vi "Convert_UI_Laundry_ERD.vi"(0 "New Header?":bool, 2 "ERD Name":string[](array[string]), 5 "All_ERD_Data_Bundled_Brass In":T1, 7 "Array":T14[](array[typedef]) {"ERD Number" format="%.0x"}, 11 "Error In":errorcluster) -> (6 "All_ERD_Data_Bundled_Brass":T1, 15 "Error Out":errorcluster)   [LabVIEW 2021]
doc: "This VI parses the data from ERDs in correct format, units, etc. It handles all hex to dec conversions, hex to enum, and hex to boolean conversions.\n\nIf Raw Data from ERD is blank string, then it will output values from shift register."
uses:
  Common/LabVIEW GEA2 Toolkit/GEA3/type defs/ERD Read Data Out.ctl
  type defs/All_Bundled_Data.ctl
  type defs/Version.ctl
  type defs/ERD_Always_Show.ctl
  type defs/Brass Matrix.ctl
  type defs/CSV_File_String_Arrays.ctl
  type defs/Redundant.ctl
  type defs/Algorithms.ctl
  type defs/ATC_Data.ctl
  type defs/Fault Table Array.ctl
  type defs/Fault_Table_Info.ctl
  Dryer Tool (Commercial 2)/JL Dryer Tool Support/type defs/ERD_RJ45.ctl
  Dryer Tool (Commercial 2)/JL Dryer Tool Support/type defs/ERD_Commercial_Laundry.ctl
  type defs/BootloaderVersion.ctl
panel:
  out "ERD Number":u16 format="%x"
  # "Wet Load Size"
  # "Dry Load Size"
  # "OOB"
  # "Wet Load Size"
  # "Dry Load Size"
  # "OOB"
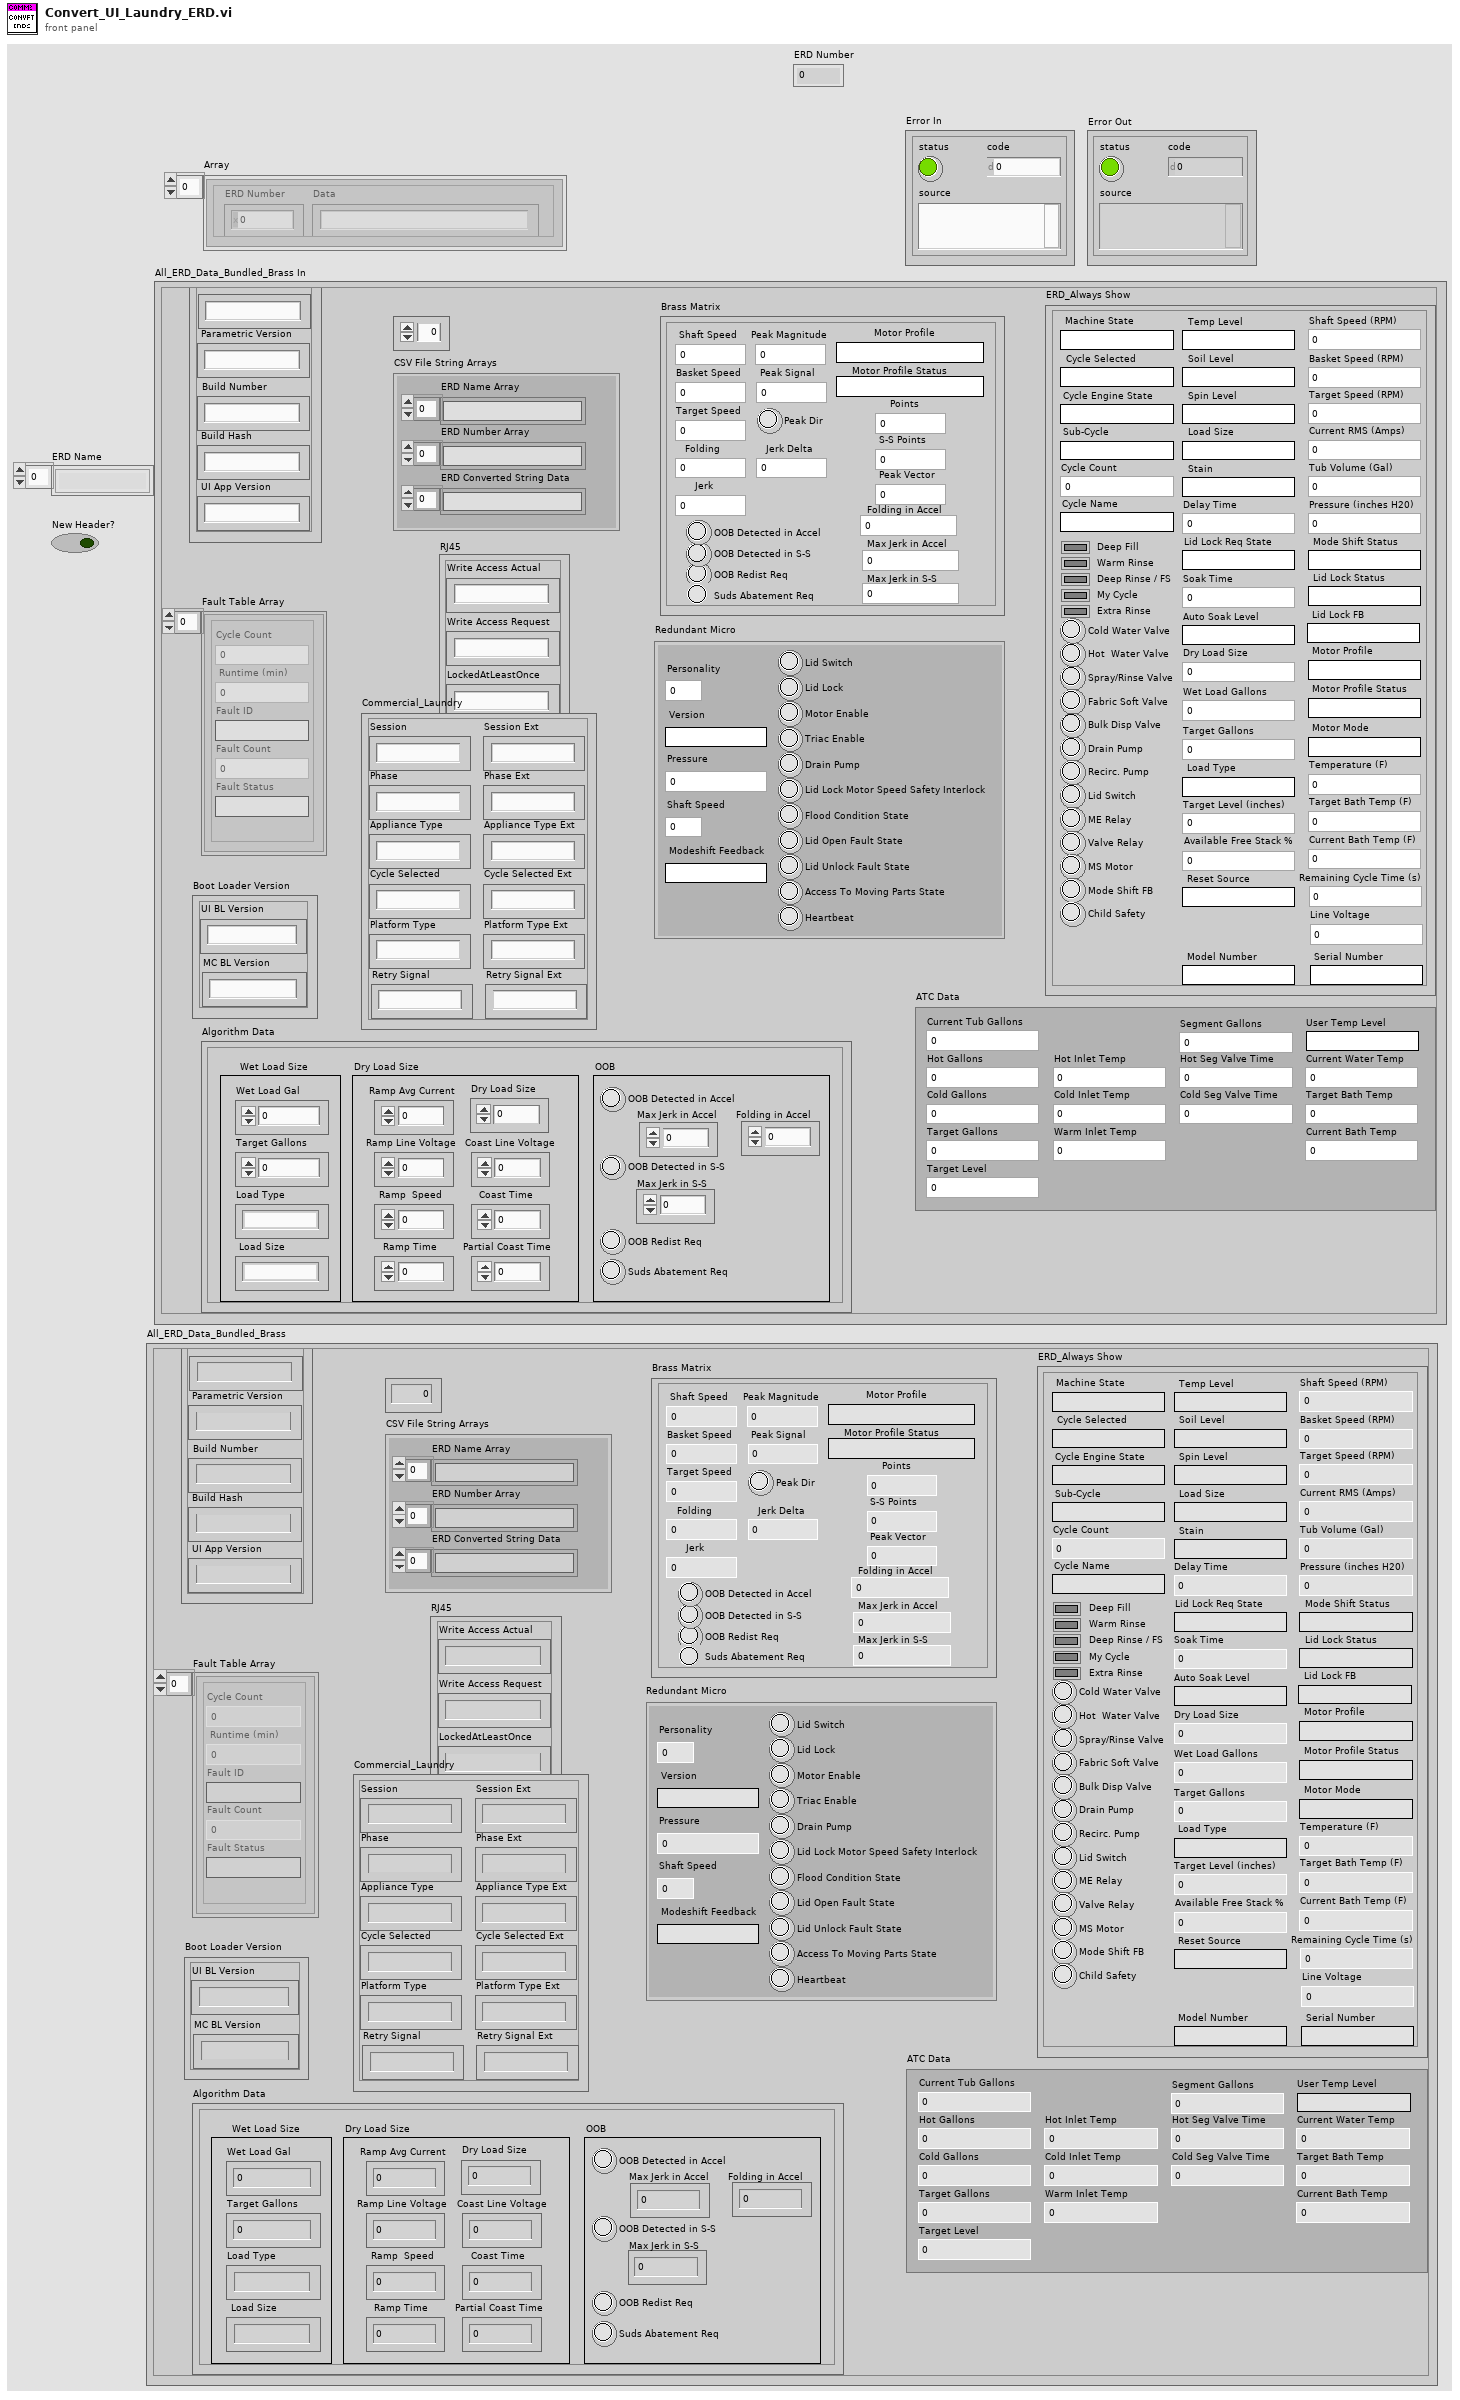
[diagram p1: front panel]
types:
  T1 = typedef "All_Bundled_Data.ctl" = cluster{"Software MC":T2, "ERD_Always Show":T3, "Personality Set":u8, "Brass Matrix":T4, "CSV File String Arrays":T5, "Redundant Micro":T6, "Algorithm Data":T7, "ATC Data":T8, "Fault Table Array ":T9, "RJ45":T11, "Commercial_Laundry":T12, "Boot Loader Version":T13}
  T2 = typedef "Version.ctl" = cluster{"Build Number":string, "Build Hash ":string, "Application Version":string, "Parametric Version":string, "UI App Version":string}
  T3 = typedef "ERD_Always_Show.ctl" = cluster{"Basket Speed (RPM)":u16, "Machine State":string, "Tub Volume (Gal)":dbl, "Pressure (inches H20)":dbl, "Lid Switch ":bool, "Current RMS (Amps)":dbl, "Cycle Selected":string, "Lid Lock Status":string, "Mode Shift Status":string, "Spray/Rinse Valve":bool, "Fabric Soft Valve":bool, "Drain Pump":bool, "Recirc. Pump":bool, "Cycle Engine State":string, "Hot  Water Valve":bool, "Cold Water Valve":bool, "Motor Profile":string, "Motor Profile Status":string, "Motor Mode":string, "ME Relay":bool, "Cycle Count":u32, "Deep Rinse / FS":bool, "My Cycle":bool, "Soil Level":string, "Spin Level":string, "Stain":string, "Temp Level":string, "Load Size":string, "Delay Time":u16, "Soak Time":u16, "Deep Fill":bool, "Warm Rinse":bool, "Auto Soak Level":string, "Extra Rinse":bool, "Wet Load Gallons":dbl, "Target Gallons":dbl, "Sub-Cycle":string, "Load Type":string, "Target Level (inches)":dbl, "Valve Relay":bool, "Dry Load Size":dbl, "Shaft Speed (RPM) ":u16, "MS Motor":bool, "Mode Shift FB":bool, "Target Bath Temp (F)":dbl, "Temperature (F)":dbl, "Current Bath Temp (F)":dbl, "Lid Lock FB":string, "Lid Lock Req State":string, "Remaining Cycle Time (s)":u32, "Available Free Stack %":u8, "Child Safety":bool, "Target Speed (RPM)":u16, "Reset Source":string, "Line Voltage":dbl, "Cycle Name":string, "Bulk Disp Valve":bool, "Model Number":string, "Serial Number":string}
  T4 = typedef "Brass Matrix.ctl" = cluster{"Shaft Speed":u16, "Folding":i32, "Jerk":i32, "Basket Speed":u16, "Target Speed":u16, "Peak Signal":u8, " Peak Magnitude":dbl, "Folding in Accel":i32, "Max Jerk in Accel":i32, "Max Jerk in S-S":i32, "Motor Profile Status":string, "Motor Profile":string, "OOB Redist Req":bool, "OOB Detected in S-S":bool, "OOB Detected in Accel":bool, "Suds Abatement Req ":bool, "Peak Dir":bool, "Peak Vector":dbl, "S-S Points":u8, "Points":u8, "Jerk Delta":i32}
  T5 = typedef "CSV_File_String_Arrays.ctl" = cluster{"ERD Number Array":string[], "ERD Name Array":string[], "ERD Converted String Data":string[]}
  T6 = typedef "Redundant.ctl" = cluster{"Version":string, "Personality":u8, "Pressure ":dbl, "Shaft Speed":u16, "Modeshift Feedback":string, "Lid Switch":bool, "Lid Lock":bool, "Triac Enable":bool, "Drain Pump":bool, "Lid Lock Motor Speed Safety Interlock":bool, "Flood Condition State":bool, "Lid Open Fault State":bool, "Access To Moving Parts State":bool, "Heartbeat":bool, "Motor Enable":bool, "Lid Unlock Fault State":bool}
  T7 = typedef "Algorithms.ctl" = cluster{"Wet Load Gal":dbl, "Target Gallons":dbl, "Load Type":string, "Load Size":string, "Coast Time":u16, "Ramp Time":u16, "Ramp  Speed":u16, "Ramp Avg Current":dbl, "OOB Redist Req":bool, "OOB Detected in S-S":bool, "Folding in Accel":i32, "Max Jerk in Accel":i32, "Max Jerk in S-S":i32, "OOB Detected in Accel":bool, "Partial Coast Time":u16, "Dry Load Size":dbl, "Ramp Line Voltage ":dbl, "Coast Line Voltage":dbl, "Suds Abatement Req ":bool}
  T8 = typedef "ATC_Data.ctl" = cluster{"Current Tub Gallons":dbl, "Hot Gallons":dbl, "Cold Gallons":dbl, "Target Gallons":dbl, "Current Water Temp":dbl, "Target Level":dbl, "Target Bath Temp":dbl, "Current Bath Temp ":dbl, "Cold Inlet Temp":dbl, "Hot Inlet Temp":dbl, "Warm Inlet Temp":dbl, "Hot Seg Valve Time":u16, "Cold Seg Valve Time ":u16, "User Temp Level":string, "Segment Gallons":dbl}
  T9 = typedef "Fault Table Array.ctl" = T10[]
  T10 = typedef "Fault_Table_Info.ctl" = cluster{"Cycle Count":u32, " Runtime (min) ":u32, "Fault Status":string, "Fault ID":string, "Fault Count":u16}
  T11 = typedef "ERD_RJ45.ctl" = cluster{"Write Access Actual":string, "Write Access Request":string, "LockedAtLeastOnce":string}
  T12 = typedef "ERD_Commercial_Laundry.ctl" = cluster{"Session":string, "Phase":string, "Appliance Type":string, "Cycle Selected":string, "Platform Type":string, "Retry Signal":string, "Session Ext":string, "Phase Ext":string, "Appliance Type Ext":string, "Cycle Selected Ext":string, "Platform Type Ext":string, "Retry Signal Ext":string}
  T13 = typedef "BootloaderVersion.ctl" = cluster{"UI BL Version":string, "MC BL Version":string}
  T14 = typedef "ERD Read Data Out.ctl" = cluster{"ERD Number":u16, "Data":string}
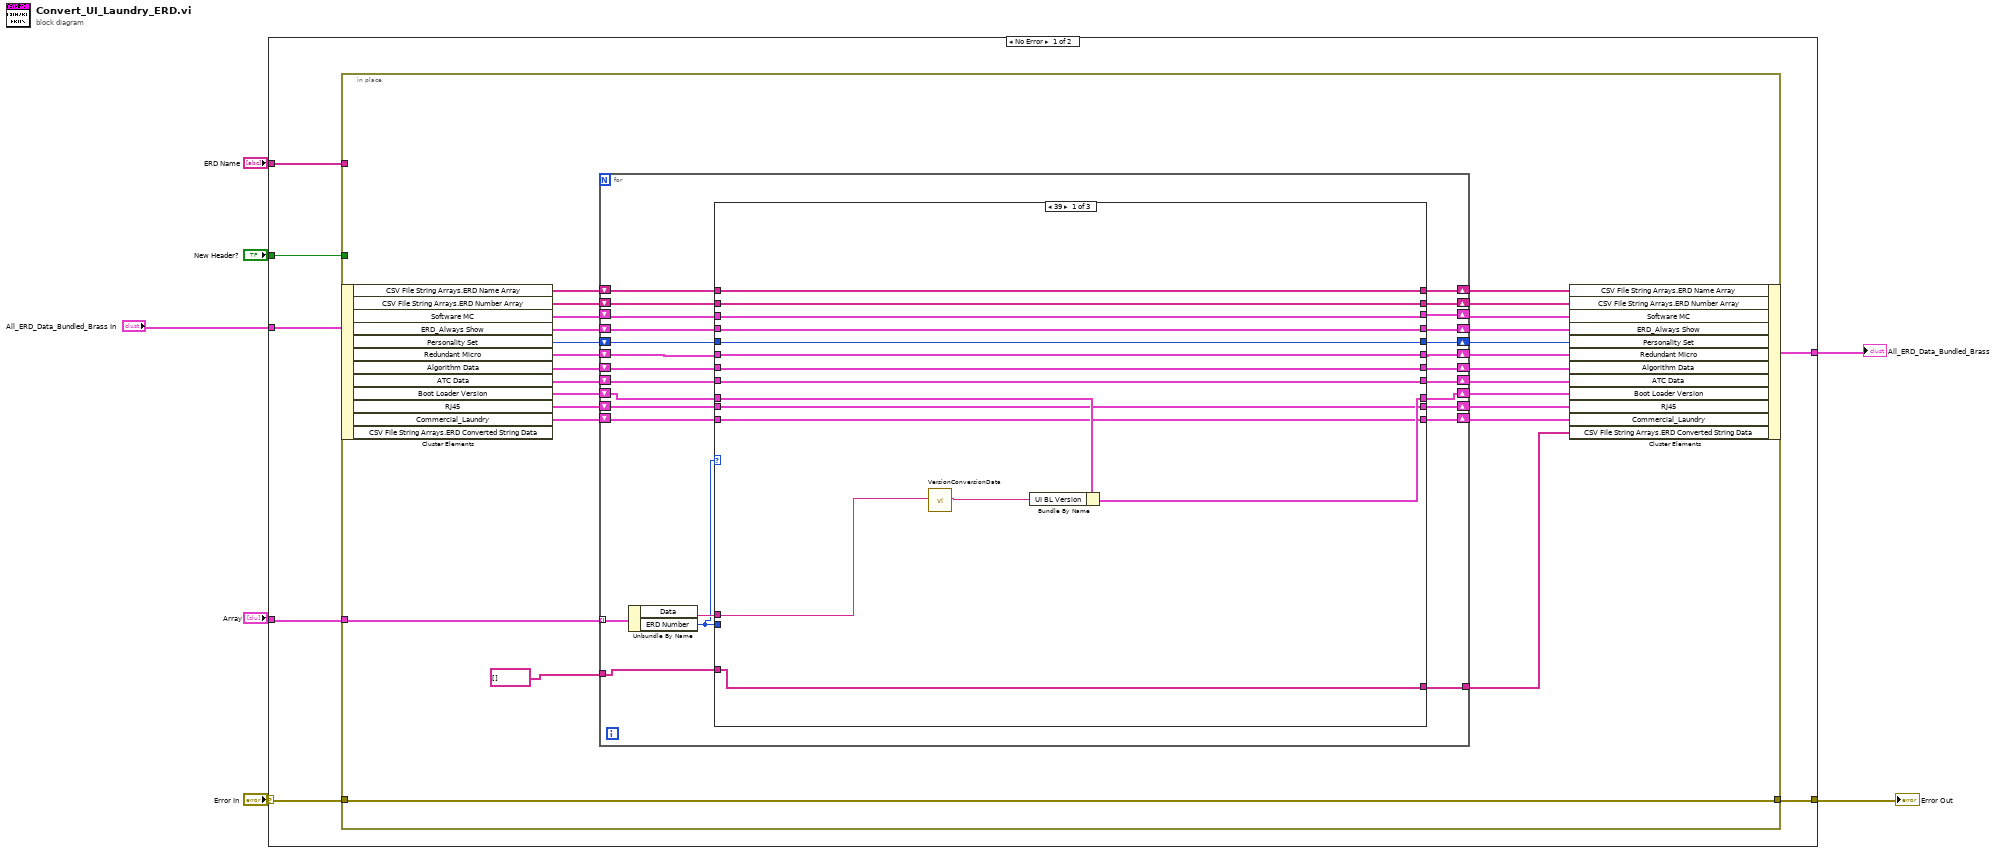
[diagram p0: block diagram]
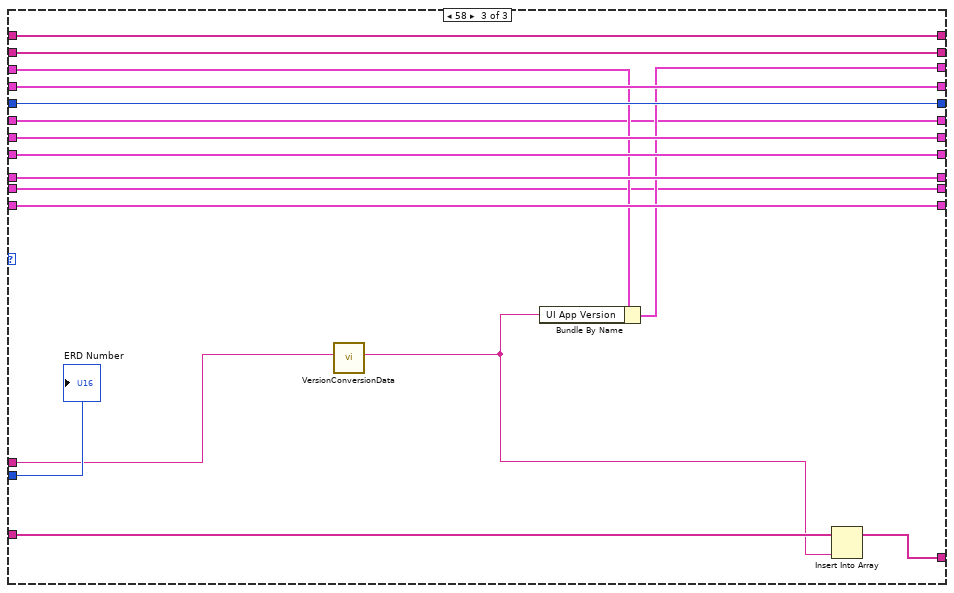
[diagram p3: hidden frame]
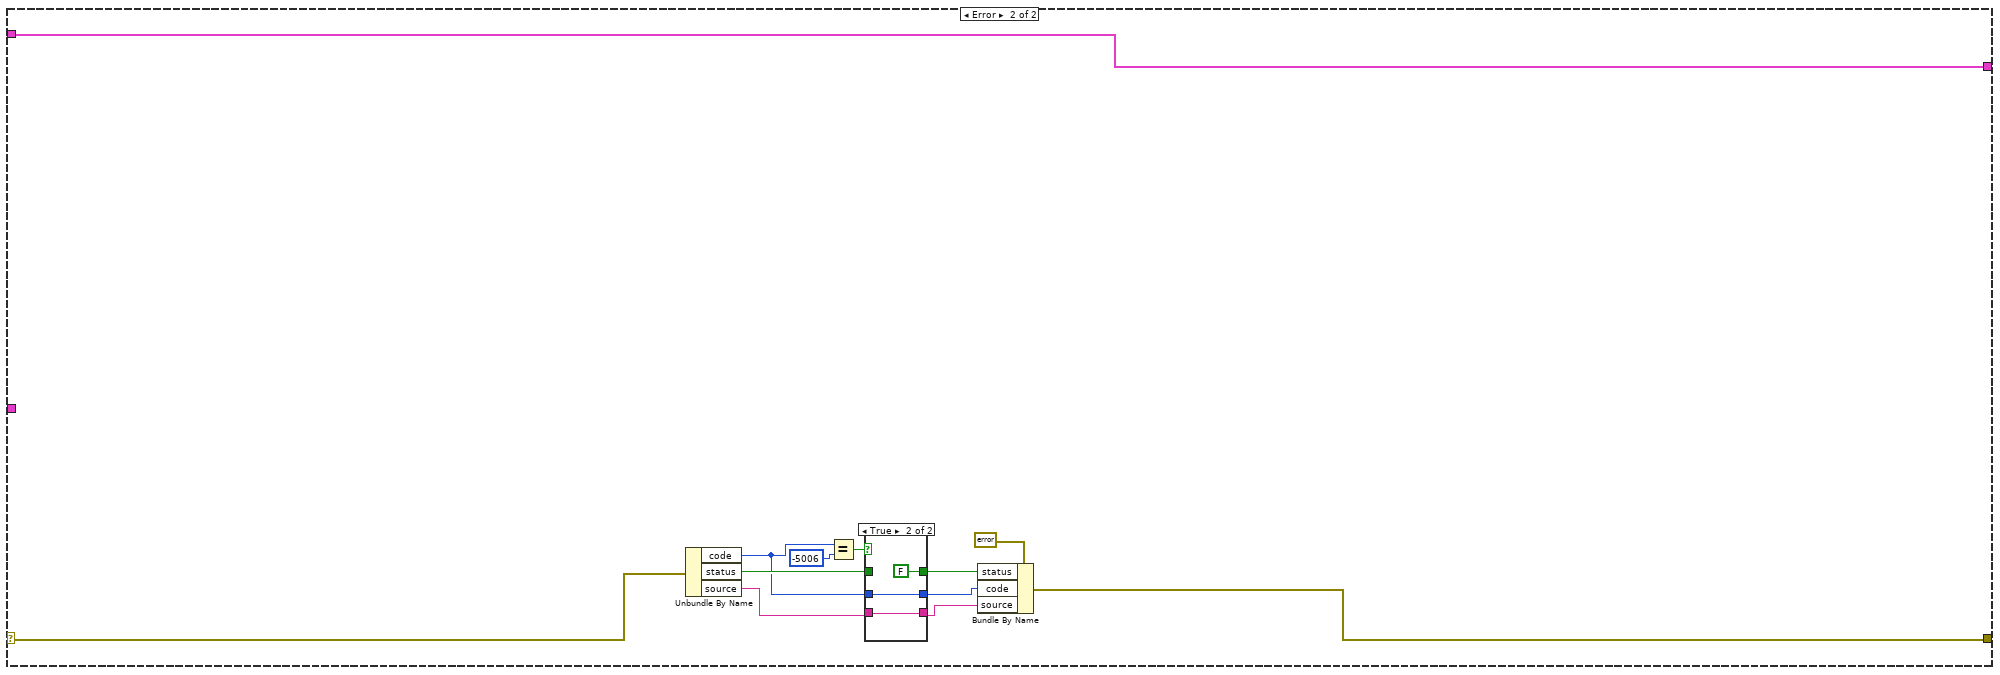
[diagram p4: hidden frame]
diagram:
  n1 = case shown="No Error" "Error In" {
    selector: "Error In" -> [w11 w114]
    tunnel: "Array" -> [w14 _]
    tunnel: [w12 w113] -> w5
    tunnel: "All_ERD_Data_Bundled_Brass In" -> [w13 w112]
    tunnel: [w10 w112] -> w1
    tunnel: "New Header?" -> [w9 _]
    tunnel: "ERD Name" -> [w8 _]
    frame No Error {
      n2 = in-place {
        in-place-border: w14 -> [w39]
        in-place-border: [w15] -> w12
        in-place-border: w11 -> [w15]
        in-place-border: w9 -> [_]
        in-place-border: w8 -> [_]
        n3 = in-place-cluster #1(w13) -> ("CSV File String Arrays.ERD Name Array"=w25:string[], "CSV File String Arrays.ERD Number Array"=w24:string[], "Software MC"=w27:T2, "ERD_Always Show"=w28:T3, "Personality Set"=w30:u8, "Redundant Micro"=w17:T6, "Algorithm Data"=w32:T7, "ATC Data"=w34:T8, "Boot Loader Version"=w37:T13, "RJ45"=w21:T11, "Commercial_Laundry"=w35:T12)  [unwired: 1 out]
        n4 = for {
          tunnel: string[] [] ("ERD String Data") -> [w64]
          tunnel: [w67] -> w18
          tunnel: w39 -> [w65] mode=indexing
          shift-right: [w61] -> w38
          shift-left: w37 -> [w62]
          shift-right: [w60] -> w36
          shift-left: w35 -> [w59]
          shift-right: [w57] -> w33
          shift-left: w34 -> [w58]
          shift-right: [w55] -> w31
          shift-left: w32 -> [w56]
          shift-right: [w48] -> w26
          shift-left: w25 -> [w47]
          shift-right: [w45] -> w23
          shift-left: w24 -> [w46]
          shift-right: [w49] -> w19
          shift-left: w27 -> [w50]
          shift-right: [w51] -> w22
          shift-left: w28 -> [w52]
          shift-right: [w53] -> w29
          shift-left: w30 -> [w54]
          shift-right: [w43] -> w20
          shift-left: w21 -> [w44]
          shift-right: [w41] -> w16
          shift-left: w17 -> [w42]
          n5 = Unbundle By Name(w65) -> ("Data"=w66:string, "ERD Number"=w63:u16)
          n6 = case shown="39" w63 {
            tunnel: [w82 w93 w111] -> w67
            tunnel: w66 -> [w70 _ w97]
            tunnel: w63 -> [_ _ w110]
            tunnel: w64 -> [w82 w93 w109]
            tunnel: w62 -> [w81 w94 w101]
            tunnel: [w80 w94 w101] -> w61
            tunnel: [w79 w85 w102] -> w60
            tunnel: w59 -> [w79 w85 w102]
            tunnel: w58 -> [w78 w86 w103]
            tunnel: [w78 w86 w103] -> w57
            tunnel: w56 -> [w77 w87 w104]
            tunnel: [w77 w87 w104] -> w55
            tunnel: w54 -> [w76 w88 w105]
            tunnel: [w76 w88 w105] -> w53
            tunnel: w52 -> [w75 w89 w106]
            tunnel: [w75 w89 w106] -> w51
            tunnel: w50 -> [w74 w90 w100]
            tunnel: [w74 w90 w99] -> w49
            tunnel: [w73 w92 w108] -> w48
            tunnel: w47 -> [w73 w92 w108]
            tunnel: w46 -> [w72 w91 w107]
            tunnel: [w72 w91 w107] -> w45
            tunnel: w44 -> [w71 w84 w98]
            tunnel: [w71 w84 w98] -> w43
            tunnel: w42 -> [w68 w83 w95]
            tunnel: [w68 w83 w95] -> w41
            frame 57 {
              n7 = call "VersionConversionData.vi"("Version In"=w70) -> ("Version Out"=w69:string)  [unwired: 9 in, 1 out]
              n8 = Bundle By Name(cluster=w81, "UI BL Version"=w69) -> (w80:T13)
            }
            frame 59, Default {
            }
            frame 58 {
              n9 = call "VersionConversionData.vi"("Version In"=w97) -> ("Version Out"=w96:string)  [unwired: 9 in, 1 out]
              n10 = Bundle By Name(cluster=w100, "UI App Version"=w96) -> (w99:T2)
              n11 = Insert Into Array(array=w109, new element=w96) -> (w111:string[])  [unwired: 1 in]
              "ERD Number" <- w110
            }
          }
        }
        n12 = in-place-cluster #1("CSV File String Arrays.ERD Name Array"=w26, "CSV File String Arrays.ERD Number Array"=w23, "Software MC"=w19, "ERD_Always Show"=w22, "Personality Set"=w29, "Redundant Micro"=w16, "Algorithm Data"=w31, "ATC Data"=w33, "Boot Loader Version"=w38, "RJ45"=w20, "Commercial_Laundry"=w36, "CSV File String Arrays.ERD Converted String Data"=w18) -> (w10:T1)
      }
    }
    frame Error {
      n13 = Unbundle By Name(w114) -> ("code"=w118:i32, "status"=w119:bool, "source"=w116:string)
      n14 = Equal?(x=w118, y=-5006) -> (x = y?=w122:bool)
      n15 = case shown="True" w122 {
        tunnel: [w126 FALSE] -> w120
        tunnel: w119 -> [w126 _]
        tunnel: w118 -> [w125 w128]
        tunnel: [w125 w128] -> w117
        tunnel: [w124 w127] -> w115
        tunnel: w116 -> [w124 w127]
        frame False {
        }
        frame True {
        }
      }
      n16 = Bundle By Name(cluster=errorcluster {"status"=FALSE, "code"=0, "source"=""} ("error constant"), "status"=w120, "code"=w117, "source"=w115) -> (w113:errorcluster)
    }
  }
  "Error Out" <- w5
  "All_ERD_Data_Bundled_Brass" <- w1
